vi "Teleop.vi"(10 "Match Info":T1={"Autonomous Elapsed Seconds"=0.0, "TeleOp Elapsed Seconds"=0.0, "Disabled Elapsed Seconds"=0.0, "Visited Autonomous"=FALSE, "Visited TeleOp"=FALSE, "Visited Disabled"=FALSE, "Autonomous Settings"={"Autonomous Style"=enum."Independent", "VI Refnum"=refnum}}, 11 "Call Context":T2) -> ()   [LabVIEW 2016]
doc: "This VI is called for each TeleOp packet received from the DS where the robot is not disabled. It is often used to read from the joysticks and update I/O or to update setpoints for timed control loops. It should complete and return within 20 milliseconds or it may miss DS packets."
uses:
  <vilib>/Rock Robotics/WPI/DriverStation/WPI_DriverStationDerivedRobotMode.ctl
  <vilib>/Rock Robotics/WPI/DriverStation/WPI_DriverStationMatch Info.ctl
  <vilib>/Rock Robotics/WPI/Utilities/WPI_GetSetVariantRefNum.vi
  <vilib>/Rock Robotics/Network Tables/NT Write Boolean Array.vi
  <vilib>/Rock Robotics/Network Tables/NT Write Numeric Array.vi
  Robot Global Data.vi
  <vilib>/functionblocks/Counter/Pulse Timer/Pulse Timer.vi
  <vilib>/Rock Robotics/WPI/Solenoid/Deprecated/WPI_SolenoidSetBool.vi
  <vilib>/functionblocks/Counter/Timer Off Delay/Timer Off Delay.vi
  <vilib>/Rock Robotics/WPI/Joystick/WPI_JoystickMecanumCartesianMapping.vi
  <vilib>/functionblocks/FB Core/FB Core.xnode
  <vilib>/functionblocks/NI_FunctionBlock Libraries.lvlib
panel:
  out "buttony":bool
  out "Servo Angle":dbl
  out "Dumper Limit Switch Top":bool
  out "Open":bool
  out "Closed":bool
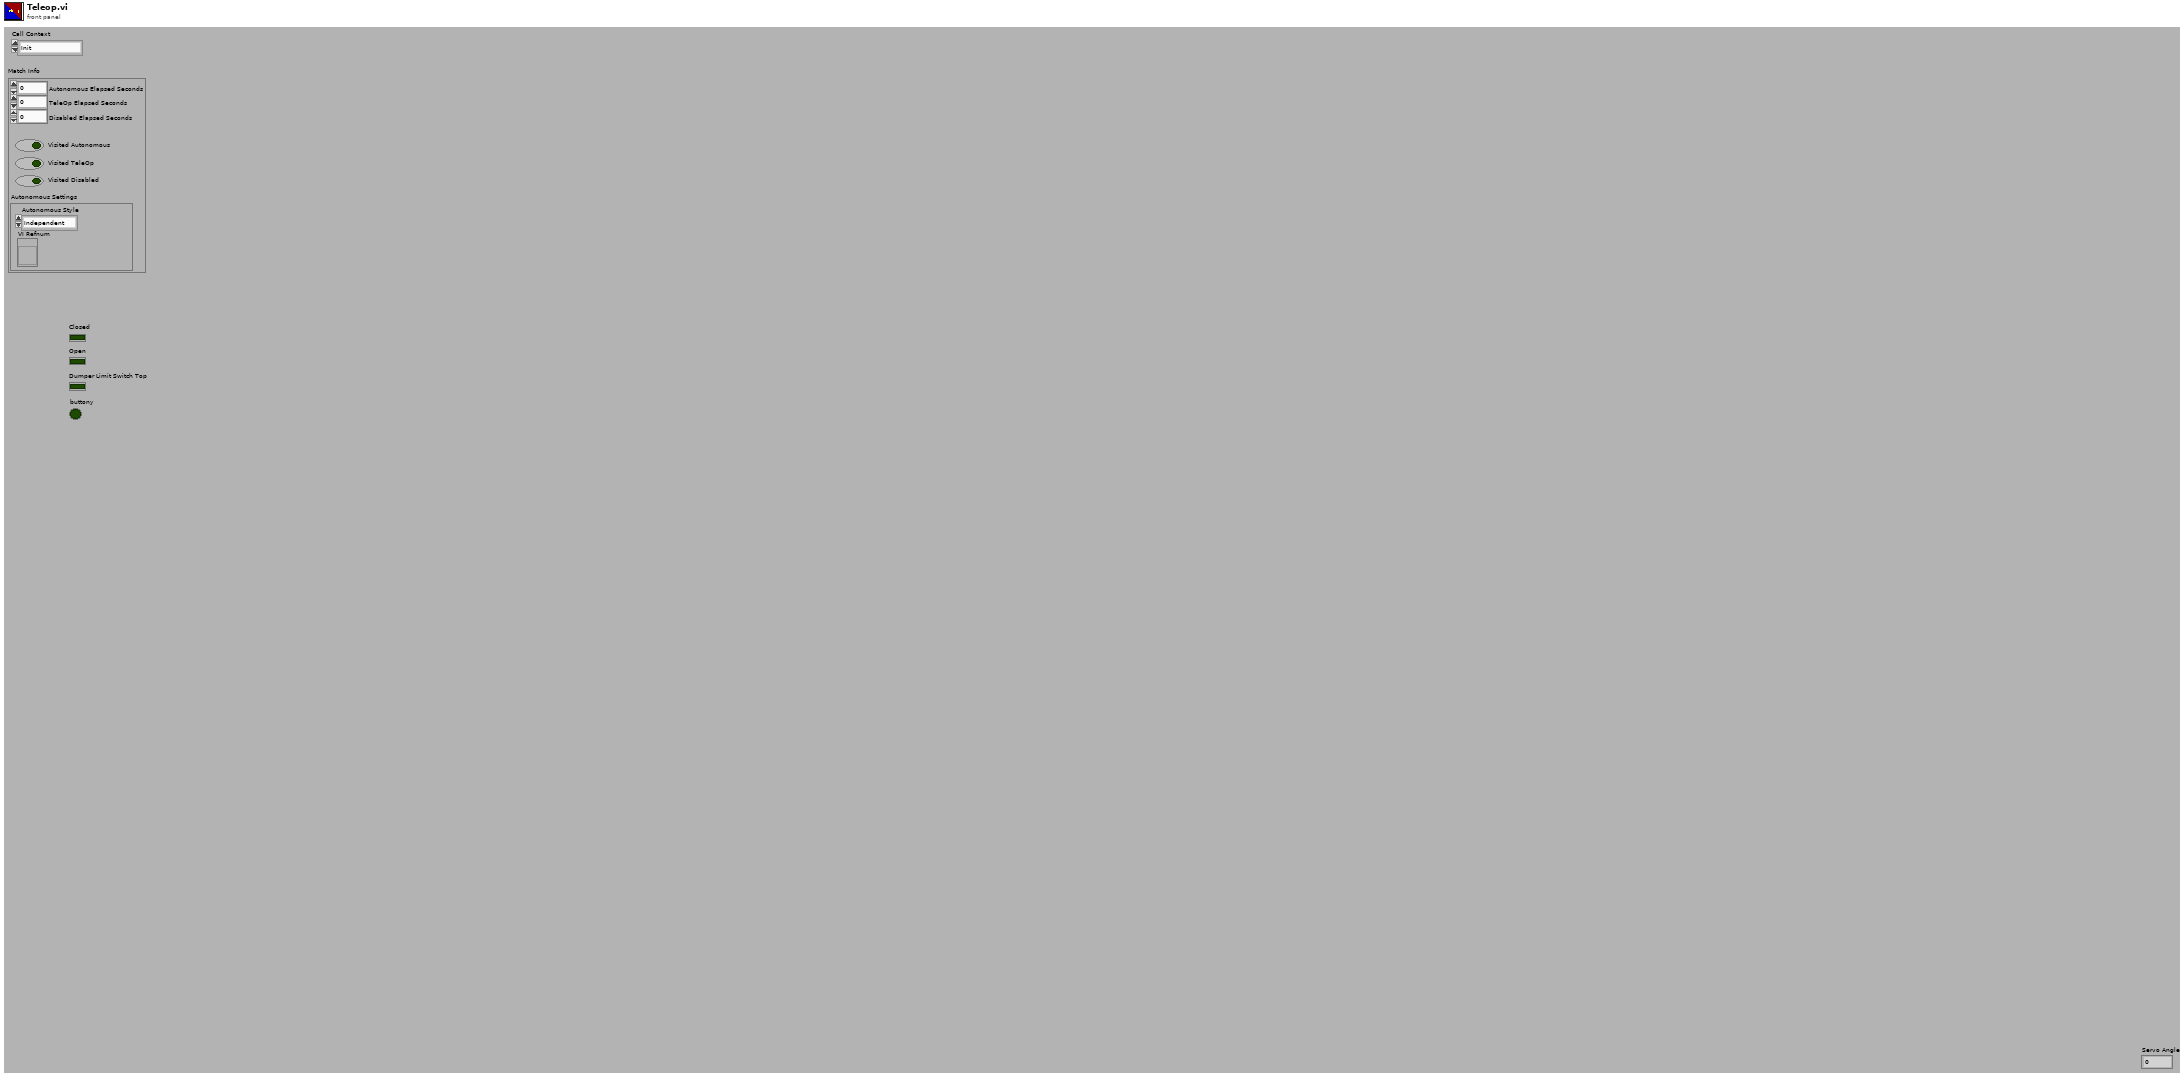
[diagram p1: front panel]
types:
  T1 = typedef "WPI_DriverStationMatch Info.ctl" = cluster{"Autonomous Elapsed Seconds":dbl, "TeleOp Elapsed Seconds":dbl, "Disabled Elapsed Seconds":dbl, "Visited Autonomous":bool, "Visited TeleOp":bool, "Visited Disabled":bool, "Autonomous Settings":cluster{"Autonomous Style":enum16{"Iterative", "Independent"}, "VI Refnum":refnum<vi>}}
  T2 = typedef "WPI_DriverStationDerivedRobotMode.ctl" = enum16{"Init", "Execute", "Stop"}
  T3 = typedef "WPI_JoystickDevRef.ctl" = cluster{"Device":T4}
  T4 = typedef "WPI_JoystickDeviceEnum.ctl" = enum16{"USB 0", "USB 1", "USB 2", "USB 3", "USB 4", "USB 5"}
  T5 = typedef "WPI_MotorControlDeviceRef.ctl" = cluster{"DeviceStatus":errorcluster, "Type":T6, "PWM":cluster{"PWM Channel":T7, "DeadBand":T8}, "CAN":cluster{"Device Number":u8, "SetOutput VI Ref":variant, "GetOutput VI Ref":variant, "Enable VI Ref":variant, "Disable VI Ref":variant, "Data":variant}, "Invert":bool}
  T6 = typedef "WPI_MotorControlType.ctl" = enum16{"PWM", "CAN"}
  T7 = typedef "FPGA_DIOPWMChannel.ctl" = enum8{"PWM 0", "PWM 1", "PWM 2", "PWM 3", "PWM 4", "PWM 5", "PWM 6", "PWM 7", "PWM 8", "PWM 9", "PWM MXP 0", "PWM MXP 1", "PWM MXP 2", "PWM MXP 3", "PWM MXP 4", "PWM MXP 5", "PWM MXP 6", "PWM MXP 7", "PWM MXP 8", "PWM MXP 9", "Invalid"}
  T8 = typedef "WPI_PWMDeadband.ctl" = cluster{"Name":string, "maxPositivePwm":i32, "minPositivePwm":i32, "centerPwm":i32, "maxNegativePwm":i32, "minNegativePwm":i32, "angularRange":u16}
  T9 = typedef "WPI_SwitchDevRef.ctl" = cluster{"DevStatus":errorcluster, "DIO Channel":T10, "CntIndex":T11, "Normally Closed":bool}
  T10 = typedef "FPGA_DIOChannel.ctl" = enum8{"DIO 0", "DIO 1", "DIO 2", "DIO 3", "DIO 4", "DIO 5", "DIO 6", "DIO 7", "DIO 8", "DIO 9", "DIO MXP 0", "DIO MXP 1", "DIO MXP 2", "DIO MXP 3", "DIO MXP 4", "DIO MXP 5", "DIO MXP 6", "DIO MXP 7", "DIO MXP 8", "DIO MXP 9", "DIO MXP 10", "DIO MXP 11", "DIO MXP 12", "DIO MXP 13", "DIO MXP 14", "DIO MXP 15", "SPI Port CS1", "SPI Port CS2", "SPI Port CS3", "SPI Port MISO", "SPI Port MOSI", "Invalid"}
  T11 = typedef "FPGA_CounterCtrSystemIndex.ctl" = enum8{"Ctr 0", "Ctr 1", "Ctr 2", "Ctr 3", "Ctr 4", "Ctr 5", "Ctr 6", "Ctr 7", "Invalid"}
  T12 = typedef "WPI_SolenoidDevRef.ctl" = cluster{"DevStatus":errorcluster, "Pneumatics Control Module":u8, "Forward Solenoid Channel":T13, "Reverse Solenoid Channel":T13}
  T13 = typedef "WPI_SolenoidChannel.ctl" = enum8{"Solenoid 0", "Solenoid 1", "Solenoid 2", "Solenoid 3", "Solenoid 4", "Solenoid 5", "Solenoid 6", "Solenoid 7", "Invalid"}
  T14 = typedef "WPI_ServoDeviceRef.ctl" = cluster{"DeviceStatus":errorcluster, "PWM Channel":T7, "DeadBand":T8}
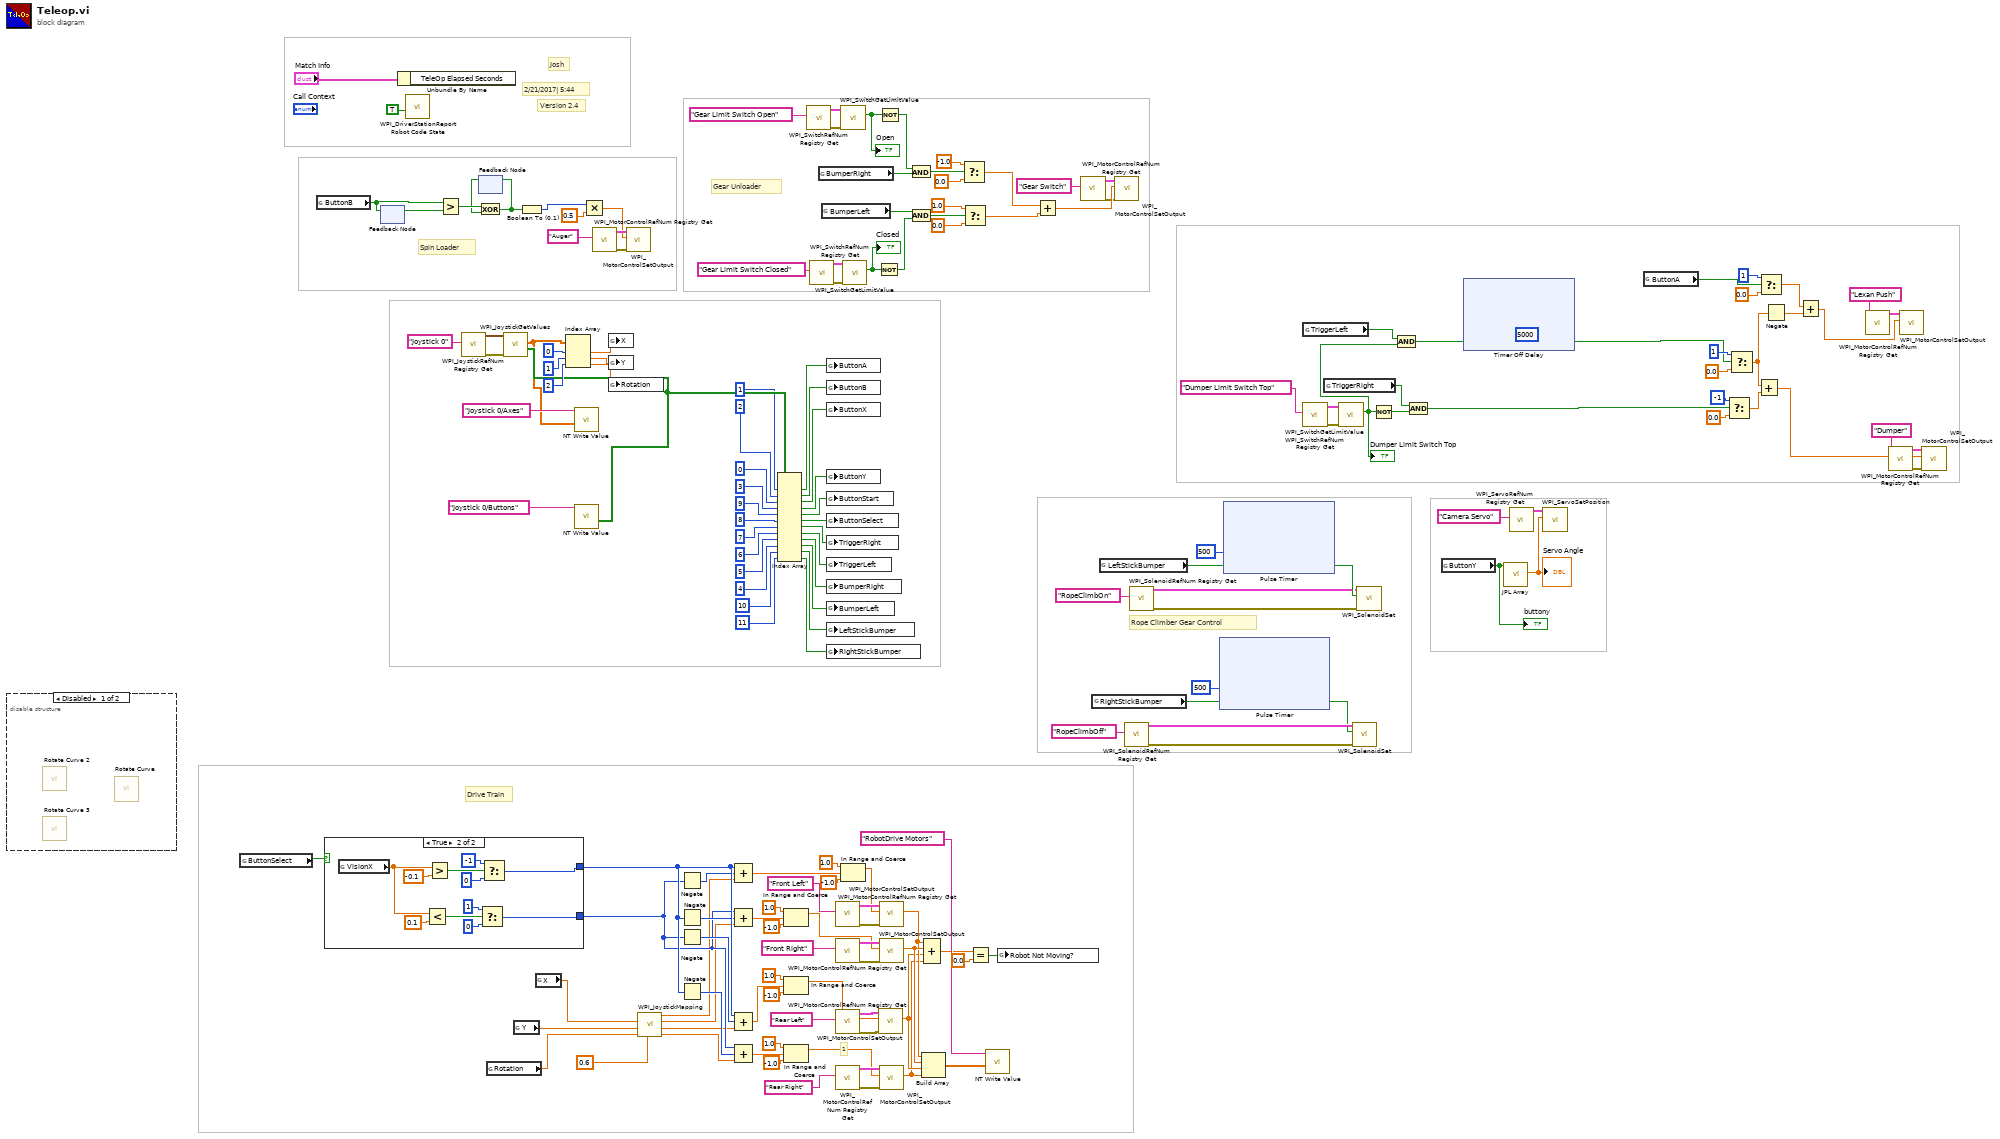
[diagram p0: block diagram]
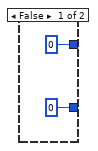
[diagram p2: hidden frame]
diagram:
  # "1"
  # "Drive Train"
  # "Josh"
  # "Rope Climber Gear Control"
  # "Gear Unloader"
  # "Spin Loader"
  # "Version 2.4"
  # "2/21/2017| 5:44"
  n1 = disable-structure shown="Disabled" {
    frame Disabled {
      n2 = call "Rotate Curve 2"() -> ()  [unwired: 10 in, 2 out]
      n3 = call "Rotate Curve 3"() -> ()  [unwired: 10 in, 2 out]
      n4 = call "Rotate Curve"() -> ()  [unwired: 10 in, 2 out]
    }
    frame Enabled {
    }
  }
  n5 = global read "Robot Global Data.vi" "ButtonSelect"() -> (w10:bool)
  n6 = global read "Robot Global Data.vi" "ButtonB"() -> (w155:bool)
  n7 = case shown="True" w10 {
    tunnel: [0 w175] -> w32
    tunnel: [0 w174] -> w34
    frame False {
    }
    frame True {
      n8 = global read "Robot Global Data.vi" "VisionX"() -> (w176:dbl)
      n9 = Less?(x=w176, y=0.1) -> (x < y?=w177:bool)
      n10 = Greater?(x=w176, y=-0.1) -> (0:w178:bool)
      n11 = Select(t=1, s=w177, f=0) -> (s? t:f=w175:i32)
      n12 = Select(t=-1, s=w178, f=0) -> (s? t:f=w174:i32)
    }
  }
  n13 = feedback #1() -> (w156:bool)  [unwired: 1 in]
  n14 = feedback-in #1(w155) -> ()
  n15 = Unbundle By Name("Match Info") -> ()  [unwired: 1 out]
  n16 = call <vilib>:"WPI_DriverStationReport Robot Code State.vi"("TeleOp"=TRUE ("Autonomous")) -> ()  [unwired: 10 in, 1 out]
  n17 = Greater?(x=w155, y=w156) -> (0:w159:bool)
  n18 = call <vilib>:"WPI_JoystickRefNum Registry Get.vi"("refnum name"="Joystick 0") -> ("error out"=w85:errorcluster, "JoystickDevRef"=w169:T3)  [unwired: 1 in, 8 out]
  n19 = feedback #2() -> (w157:bool)  [unwired: 1 in]
  n20 = Exclusive Or(1:w157, 2:w159) -> (0:w158:bool)
  n21 = feedback-in #2(w158) -> ()
  n22 = global read "Robot Global Data.vi" "Rotation"() -> (w7:dbl)
  n23 = call <vilib>:"WPI_JoystickGetValues.vi"("error in (no error)"=w85, "JoystickDevRef"=w169) -> ("Buttons"=w127:bool[], "Axes"=w117:dbl[])  [unwired: 5 in, 3 out]
  n24 = global read "Robot Global Data.vi" "Y"() -> (w8:dbl)
  n25 = Boolean To (0,1)(Boolean=w158) -> (0, 1=w70:i16)
  n26 = global read "Robot Global Data.vi" "X"() -> (w9:dbl)
  n27 = Index Array(array=w117, index #1=0, index #2=1, index #3=2) -> (element #1=w162:dbl, element #2=w160:dbl, element #3=w161:dbl)
  n28 = call-poly <vilib>:"NT Write Value.vi"("Numeric Array"=w117, "Name"="Joystick 0/Axes") -> ()  [unwired: 9 in, 1 out]
  n29 = call-poly <vilib>:"NT Write Value.vi"("Boolean Array"=w127, "Name"="Joystick 0/Buttons") -> ()  [unwired: 9 in, 1 out]
  n30 = Multiply(x=w70, y=0.5) -> (x*y=w69:dbl)
  n31 = call <vilib>:"WPI_MotorControlRefNum Registry Get.vi"("refnum name"="Auger") -> ("error out"=w118:errorcluster, "MotorControlDevRef"=w116:T5)  [unwired: 9 in]
  n32 = global write "Robot Global Data.vi" "X"(w162) -> ()
  n33 = global write "Robot Global Data.vi" "Y"(w160) -> ()
  n34 = global write "Robot Global Data.vi" "Rotation"(w161) -> ()
  n35 = call <vilib>:"WPI_MotorControlSetOutput.vi"("error in (no error)"=w118, "Output"=w69, "MotorControlDevRef"=w116) -> ()  [unwired: 6 in, 3 out]
  n36 = call-poly <vilib>:"WPI_JoystickMapping.vi"("Max Output"=0.6, "Rotation"=w7, "Y"=w8, "X"=w9) -> ("Rear Right"=w28:dbl, "Rear Left"=w30:dbl, "Front Right"=w27:dbl, "Front Left"=w29:dbl)  [unwired: 4 in]
  n37 = Negate(x=w32) -> (-x=w31:i32)
  n38 = Negate(x=w34) -> (-x=w33:i32)
  n39 = Negate(x=w32) -> (-x=w36:i32)
  n40 = Negate(x=w34) -> (-x=w35:i32)
  n41 = Compound Arithmetic op=ADD(w34, w31, w29) -> (w16:dbl)
  n42 = Compound Arithmetic op=ADD(w32, w33, w27) -> (w18:dbl)
  n43 = Compound Arithmetic op=ADD(w34, w36, w30) -> (w15:dbl)
  n44 = Compound Arithmetic op=ADD(w32, w35, w28) -> (w17:dbl)
  n45 = Index Array(array=w127, index #1=1, index #2=2, index #3=0, index #4=3, index #5=9, index #6=8, index #7=7, index #8=6, index #9=5, index #10=4, index #11=10, index #12=11) -> (element #1=w130:bool, element #2=w129:bool, element #3=w128:bool, element #4=w126:bool, element #5=w125:bool, element #6=w124:bool, element #7=w123:bool, element #8=w122:bool, element #9=w121:bool, element #10=w120:bool, element #11=w114:bool, element #12=w113:bool)
  n46 = In Range and Coerce(upper limit=1.0, x=w18, lower limit=-1.0) -> (coerced(x)=w11:dbl)  [unwired: 1 out]
  n47 = In Range and Coerce(upper limit=1.0, x=w15, lower limit=-1.0) -> (coerced(x)=w14:dbl)  [unwired: 1 out]
  n48 = In Range and Coerce(upper limit=1.0, x=w17, lower limit=-1.0) -> (coerced(x)=w12:dbl)  [unwired: 1 out]
  n49 = call <vilib>:"WPI_SwitchRefNum Registry Get.vi"("refnum name"="Gear Limit Switch Open") -> ("error out"=w83:errorcluster, "SwitchDevRef"=w147:T9)  [unwired: 9 in]
  n50 = call <vilib>:"WPI_SwitchRefNum Registry Get.vi"("refnum name"="Gear Limit Switch Closed") -> ("error out"=w82:errorcluster, "SwitchDevRef"=w149:T9)  [unwired: 9 in]
  n51 = global read "Robot Global Data.vi" "BumperRight"() -> (w145:bool)
  n52 = global read "Robot Global Data.vi" "BumperLeft"() -> (w144:bool)
  n53 = global write "Robot Global Data.vi" "ButtonA"(w130) -> ()
  n54 = global write "Robot Global Data.vi" "ButtonB"(w129) -> ()
  n55 = global write "Robot Global Data.vi" "ButtonX"(w128) -> ()
  n56 = global write "Robot Global Data.vi" "ButtonY"(w126) -> ()
  n57 = global write "Robot Global Data.vi" "ButtonStart"(w125) -> ()
  n58 = global write "Robot Global Data.vi" "ButtonSelect"(w124) -> ()
  n59 = global write "Robot Global Data.vi" "TriggerRight"(w123) -> ()
  n60 = global write "Robot Global Data.vi" "TriggerLeft"(w122) -> ()
  n61 = global write "Robot Global Data.vi" "BumperRight"(w121) -> ()
  n62 = global write "Robot Global Data.vi" "BumperLeft"(w120) -> ()
  n63 = global write "Robot Global Data.vi" "LeftStickBumper"(w114) -> ()
  n64 = global write "Robot Global Data.vi" "RightStickBumper"(w113) -> ()
  n65 = call <vilib>:"WPI_MotorControlRefNum Registry Get.vi"("refnum name"="Front Left") -> ("error out"=w48:errorcluster, "MotorControlDevRef"=w53:T5)  [unwired: 9 in]
  n66 = call <vilib>:"WPI_MotorControlRefNum Registry Get.vi"("refnum name"="Front Right") -> ("error out"=w49:errorcluster, "MotorControlDevRef"=w52:T5)  [unwired: 9 in]
  n67 = call <vilib>:"WPI_MotorControlRefNum Registry Get.vi"("refnum name"="Rear Left") -> ("error out"=w47:errorcluster, "MotorControlDevRef"=w50:T5)  [unwired: 9 in]
  n68 = call <vilib>:"WPI_MotorControlRefNum Registry Get.vi"("refnum name"="Rear Right") -> ("error out"=w46:errorcluster, "MotorControlDevRef"=w51:T5)  [unwired: 9 in]
  n69 = call <vilib>:"WPI_SwitchGetLimitValue.vi"("error in (no error)"=w83, "SwitchDevRef"=w147) -> ("Switch Pressed"=w131:bool)  [unwired: 7 in, 2 out]
  "Open" <- w131
  n70 = In Range and Coerce(upper limit=1.0, x=w16, lower limit=-1.0) -> (coerced(x)=w13:dbl)  [unwired: 1 out]
  n71 = call <vilib>:"WPI_SwitchGetLimitValue.vi"("error in (no error)"=w82, "SwitchDevRef"=w149) -> ("Switch Pressed"=w134:bool)  [unwired: 7 in, 2 out]
  "Closed" <- w134
  n72 = Not(x=w134) -> (.not. x?=w133:bool)
  n73 = Not(x=w131) -> (.not. x?=w132:bool)
  n74 = call <vilib>:"WPI_MotorControlSetOutput.vi"("error in (no error)"=w47, "Output"=w14, "MotorControlDevRef"=w50) -> ("Motor Output"=w41:dbl)  [unwired: 6 in, 2 out]
  n75 = call <vilib>:"WPI_MotorControlSetOutput.vi"("error in (no error)"=w48, "Output"=w13, "MotorControlDevRef"=w53) -> ("Motor Output"=w42:dbl)  [unwired: 6 in, 2 out]
  n76 = call <vilib>:"WPI_MotorControlSetOutput.vi"("error in (no error)"=w49, "Output"=w11, "MotorControlDevRef"=w52) -> ("Motor Output"=w43:dbl)  [unwired: 6 in, 2 out]
  n77 = call <vilib>:"WPI_MotorControlSetOutput.vi"("error in (no error)"=w46, "Output"=w12, "MotorControlDevRef"=w51) -> ("Motor Output"=w40:dbl)  [unwired: 6 in, 2 out]
  n78 = And(x=w132, y=w145) -> (x .and. y?=w136:bool)
  n79 = And(x=w144, y=w133) -> (x .and. y?=w135:bool)
  n80 = Build Array(w42, w43, w41, w40) -> (w45:dbl[])
  n81 = Compound Arithmetic op=ADD(w42, w43, w41, w40) -> (w38:dbl)
  n82 = Select(t=-1.0, s=w136, f=0.0) -> (s? t:f=w139:dbl)
  n83 = Select(t=1.0, s=w135, f=0.0) -> (s? t:f=w138:dbl)
  n84 = Equal?(x=w38, y=0.0) -> (x = y?=w37:bool)
  n85 = call-poly <vilib>:"NT Write Value.vi"("Numeric Array"=w45, "Name"="RobotDrive Motors") -> ()  [unwired: 9 in, 1 out]
  n86 = global write "Robot Global Data.vi" "Robot Not Moving?"(w37) -> ()
  n87 = Add(x=w139, y=w138) -> (x+y=w137:dbl)
  n88 = call <vilib>:"WPI_MotorControlRefNum Registry Get.vi"("refnum name"="Gear Switch") -> ("error out"=w84:errorcluster, "MotorControlDevRef"=w150:T5)  [unwired: 9 in]
  n89 = global read "Robot Global Data.vi" "RightStickBumper"() -> (w99:bool)
  n90 = global read "Robot Global Data.vi" "LeftStickBumper"() -> (w105:bool)
  n91 = call <vilib>:"WPI_MotorControlSetOutput.vi"("error in (no error)"=w84, "Output"=w137, "MotorControlDevRef"=w150) -> ()  [unwired: 6 in, 3 out]
  n92 = call <vilib>:"WPI_SolenoidRefNum Registry Get.vi"("refnum name"="RopeClimbOff") -> ("error out"=w97:errorcluster, "SolenoidDevRef"=w101:T12)  [unwired: 9 in]
  n93 = call <vilib>:"WPI_SolenoidRefNum Registry Get.vi"("refnum name"="RopeClimbOn") -> ("error out"=w115:errorcluster, "SolenoidDevRef"=w103:T12)  [unwired: 9 in]
  n94 = xnode "Pulse Timer"("preset time (ms)"=500, "input"=w99) -> ("output"=w98:bool)  [unwired: 1 in, 2 out]
  n95 = xnode "Pulse Timer"("preset time (ms)"=500, "input"=w105) -> ("output"=w104:bool)  [unwired: 1 in, 2 out]
  n96 = global read "Robot Global Data.vi" "TriggerLeft"() -> (w63:bool)
  n97 = call <vilib>:"WPI_SwitchRefNum Registry Get.vi"("refnum name"="Dumper Limit Switch Top") -> ("error out"=w81:errorcluster, "SwitchDevRef"=w112:T9)  [unwired: 9 in]
  n98 = global read "Robot Global Data.vi" "TriggerRight"() -> (w110:bool)
  n99 = call <vilib>:"WPI_SwitchGetLimitValue.vi"("error in (no error)"=w81, "SwitchDevRef"=w112) -> ("Switch Pressed"=w64:bool)  [unwired: 7 in, 2 out]
  "Dumper Limit Switch Top" <- w64
  n100 = call-poly <vilib>:"WPI_SolenoidSet.vi"("error in (no error)"=w97, "Value"=w98, "SolenoidDevRef"=w101) -> ()  [unwired: 7 in, 2 out]
  n101 = call-poly <vilib>:"WPI_SolenoidSet.vi"("error in (no error)"=w115, "Value"=w104, "SolenoidDevRef"=w103) -> ()  [unwired: 7 in, 2 out]
  n102 = Not(x=w64) -> (.not. x?=w77:bool)
  n103 = And(x=w63, y=w64) -> (x .and. y?=w62:bool)
  n104 = And(x=w110, y=w77) -> (x .and. y?=w80:bool)
  n105 = global read "Robot Global Data.vi" "ButtonY"() -> (w66:bool)
  "buttony" <- w66
  n106 = xnode "Timer Off Delay"("preset time (ms)"=5000, "input"=w62) -> ("output"=w75:bool)  [unwired: 1 in, 2 out]
  n107 = call "JPL Array.vi"("Boolean"=w66) -> ("Value"=w67:dbl)  [unwired: 9 in, 1 out]
  "Servo Angle" <- w67
  n108 = call <vilib>:"WPI_ServoRefNum Registry Get.vi"("refnum name"="Camera Servo") -> ("ServoDeviceRef"=w71:T14)  [unwired: 9 in, 1 out]
  n109 = call <vilib>:"WPI_ServoSetPosition.vi"("Position"=w67, "ServoDeviceRef"=w71) -> ()  [unwired: 8 in, 2 out]
  n110 = global read "Robot Global Data.vi" "ButtonA"() -> (w59:bool)
  n111 = Select(t=-1, s=w80, f=0.0) -> (s? t:f=w76:dbl)
  n112 = Select(t=1, s=w75, f=0.0) -> (s? t:f=w5:dbl)
  n113 = Add(x=w5, y=w76) -> (x+y=w73:dbl)
  n114 = Select(t=1, s=w59, f=0.0) -> (s? t:f=w6:dbl)
  n115 = Negate(x=w5) -> (-x=w4:dbl)
  n116 = Add(x=w6, y=w4) -> (x+y=w1:dbl)
  n117 = call <vilib>:"WPI_MotorControlRefNum Registry Get.vi"("refnum name"="Lexan Push") -> ("MotorControlDevRef"=w2:T5)  [unwired: 9 in, 1 out]
  n118 = call <vilib>:"WPI_MotorControlRefNum Registry Get.vi"("refnum name"="Dumper") -> ("error out"=w154:errorcluster, "MotorControlDevRef"=w152:T5)  [unwired: 9 in]
  n119 = call <vilib>:"WPI_MotorControlSetOutput.vi"("Output"=w1, "MotorControlDevRef"=w2) -> ()  [unwired: 7 in, 3 out]
  n120 = call <vilib>:"WPI_MotorControlSetOutput.vi"("error in (no error)"=w154, "Output"=w73, "MotorControlDevRef"=w152) -> ()  [unwired: 6 in, 3 out]
